vi "44xx_AI_MinMax.vi"(9 "AI.channels":tag, 10 "446x AI":T1) -> (1 "ProductType":string, 2 "AI.Max":dbl, 3 "AI.Min":dbl)   [LabVIEW 2016, in "LockinDAQ.lvclass"]
uses:
  LockinDAQ.lvclass
  Typedefs/446xAI-enum.ctl
  <resource>/objmgr/daqmx.rc
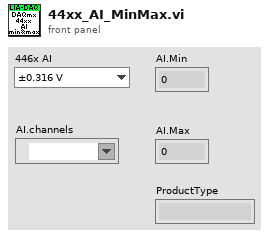
[diagram p1: front panel]
types:
  T1 = typedef "446xAI-enum.ctl" = enum16{"±0.316 V", "±1.00 V", "±3.16 V", "±10.0 V", "±31.6 V", "±42.4 V"}
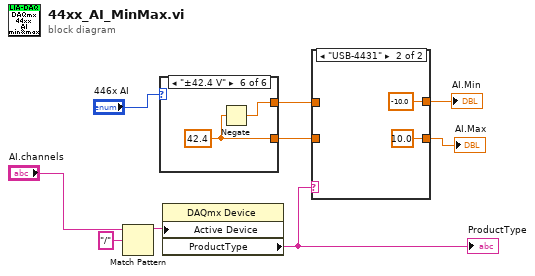
[diagram p0: block diagram]
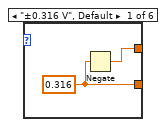
[diagram p3: hidden frame]
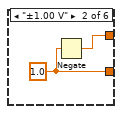
[diagram p4: hidden frame]
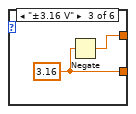
[diagram p5: hidden frame]
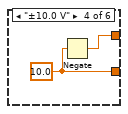
[diagram p6: hidden frame]
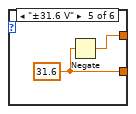
[diagram p7: hidden frame]
diagram:
  n1 = Match Pattern(string="AI.channels", regular expression="/") -> (before substring=w7:string)  [unwired: 1 in, 3 out]
  n2 = case shown="\"±42.4 V\"" "446x AI" {
    tunnel: [w10 w12 w14 w16 w18 w20] -> w3
    tunnel: [w11 w13 w15 w17 w19 w21] -> w1
    frame "±0.316 V", Default {
      w11 = 0.316 ("AI.Min")
      n3 = Negate(x=w11) -> (-x=w10:dbl)
    }
    frame "±1.00 V" {
      w13 = 1.0 ("AI.Min")
      n4 = Negate(x=w13) -> (-x=w12:dbl)
    }
    frame "±3.16 V" {
      w15 = 3.16 ("AI.Min")
      n5 = Negate(x=w15) -> (-x=w14:dbl)
    }
    frame "±10.0 V" {
      w17 = 10.0 ("AI.Min")
      n6 = Negate(x=w17) -> (-x=w16:dbl)
    }
    frame "±31.6 V" {
      w19 = 31.6 ("AI.Min")
      n7 = Negate(x=w19) -> (-x=w18:dbl)
    }
    frame "±42.4 V" {
      w21 = 42.4 ("AI.Min")
      n8 = Negate(x=w21) -> (-x=w20:dbl)
    }
  }
  n9 = property class="DAQmx Device"("Active Device"=w7) -> ("ProductType"=w5:string)  [unwired: 2 in, 2 out]
  "ProductType" <- w5
  n10 = case shown="\"USB-4431\"" w5 {
    tunnel: [w23 -10.0] -> w4
    tunnel: w3 -> [w23 _]
    tunnel: [w22 10.0 ("AI.Min")] -> w2
    tunnel: w1 -> [w22 _]
    frame "", Default {
    }
    frame "USB-4431" {
    }
  }
  "AI.Min" <- w4
  "AI.Max" <- w2
